vi "__2400_read_vi.vi"(7 "GPIB":string="24") -> (0 "error out":errorcluster caption="エラー出力", 2 "volt_current (mA)":dbl, 3 "volt_read (mV)":dbl)   [LabVIEW 2017]
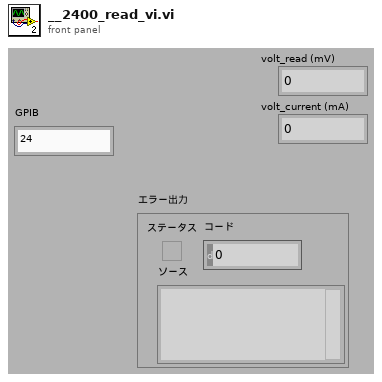
[diagram p1: front panel]
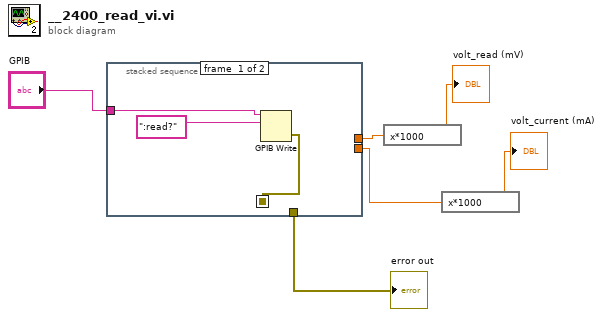
[diagram p0: block diagram]
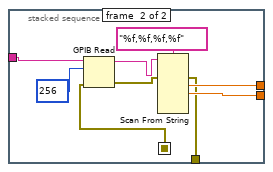
[diagram p2: hidden frame]
diagram:
  n1 = stacked-sequence {
    seq-local: [w7 _] -> [_ w12]
    tunnel: "GPIB" -> [w9 w18]
    tunnel: [_ w14] -> w5
    tunnel: [_ w13] -> w2
    tunnel: [_ w10] -> w1
    frame #0 {
      n2 = GPIB Write(0:w9, 1:":read?") -> (6:w7:errorcluster)  [unwired: 3 in, 1 out]
    }
    frame #1 {
      n3 = GPIB Read(0:w18, 1:256, 3:w12) -> (5:w16:string, 7:w11:errorcluster)  [unwired: 2 in, 1 out]
      n4 = Scan From String(format string="%f,%f,%f,%f", input string=w16, error in=w11) -> (error out=w10:errorcluster, output 1=w14:dbl, output 2=w13:dbl)  [unwired: 7 in, 2 out]
    }
  }
  "error out" <- w1
  n5 = expression code="x*1000"(w5) -> (→"volt_read (mV)":dbl)
  n6 = expression code="x*1000"(w2) -> (→"volt_current (mA)":dbl)
